vi "报警设置.vi"() -> ()   [LabVIEW 2016, in "环境动力单元.lvlib"]
uses:
  <vilib>/Utility/config.llb/NI_LVConfig.lvlib
panel:
  out "湿度报警解除阈值 %":dbl=90.0
  out "高温报警解除阈值 ℃":dbl=40.0
  out "低压报警解除阈值 V":dbl=13.0
  out "湿度报警阈值 %":dbl=95.0
  out "高温报警阈值 ℃":dbl=50.0
  out "低压报警阈值 V":dbl=11.0
  in  "布尔":bool
  # "参数设置"
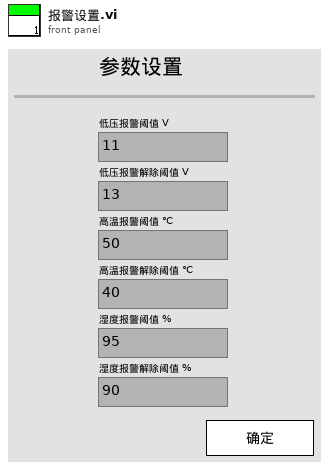
[diagram p1: front panel]
types:
  T1 = cluster{"低压报警阈值 V":dbl, "低压报警解除阈值 V":dbl, "高温报警阈值 ℃":dbl, "高温报警解除阈值 ℃":dbl, "湿度报警阈值 %":dbl, "湿度报警解除阈值 %":dbl}
  T2 = typedef "NI_LVConfig.lvlib/Config Data RefNum.ctl" = refnum<k1>
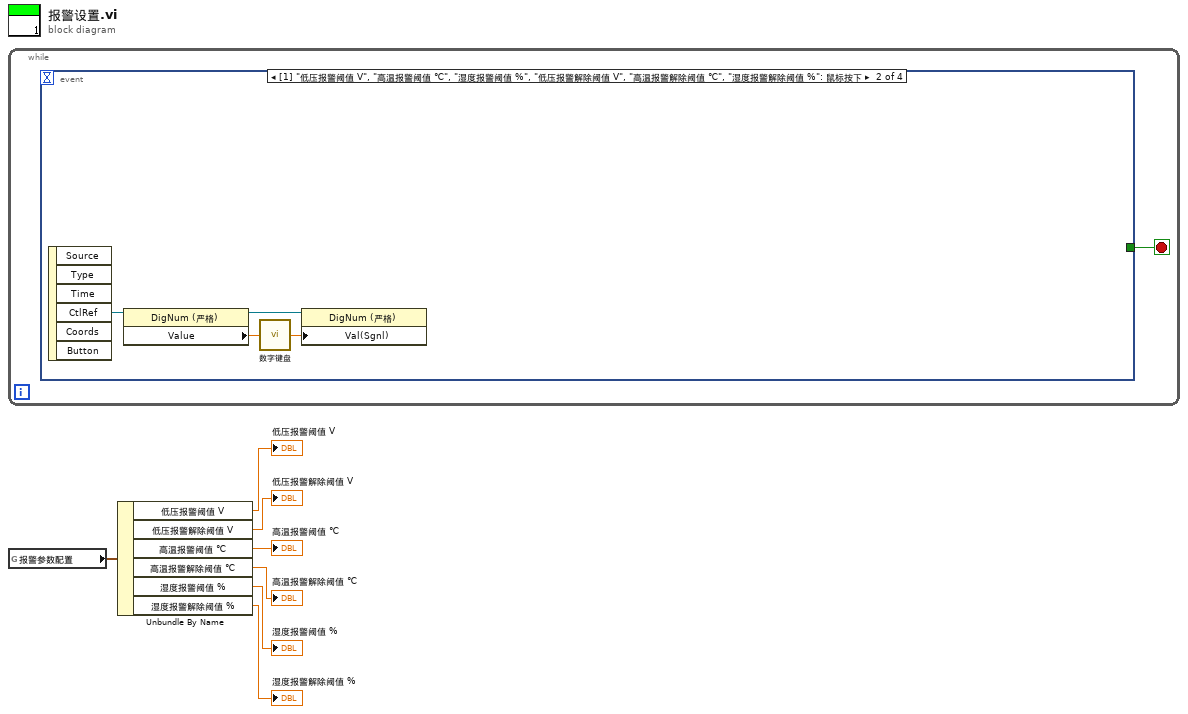
[diagram p0: block diagram]
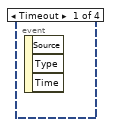
[diagram p2: hidden frame]
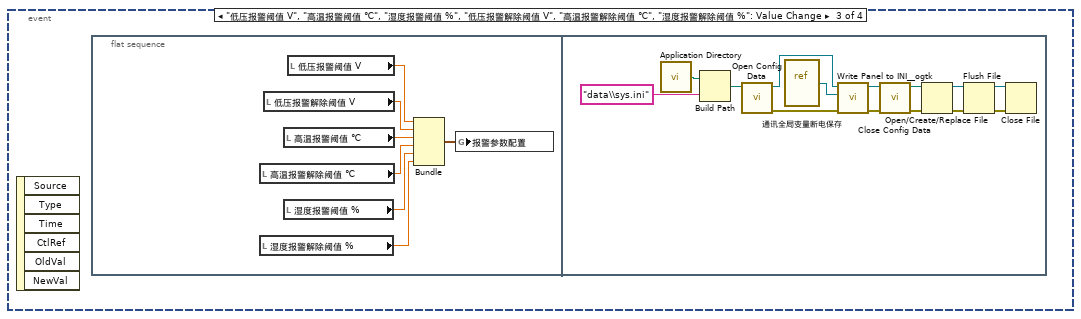
[diagram p3: hidden frame]
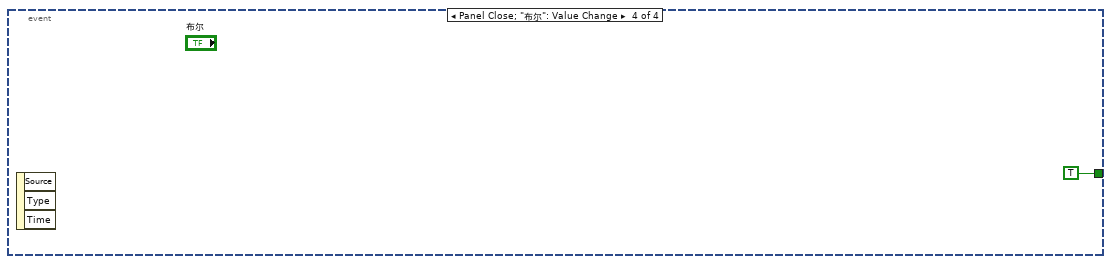
[diagram p4: hidden frame]
diagram:
  n1 = while {
    stop <- w8 stop-if-true
    n2 = event shown="[1] \"低压报警阈值 V\", \"高温报警阈值 ℃\", \"湿度报警阈值 %\", \"低压报警解除阈值 V\", \"高温报警解除阈值 ℃\", \"湿度报警解除阈值 %\": 鼠标按下" {
      selector: _ -> [_ _ _ _]
      dyn-events: _ -> [_ _ _ _]
      timeout: _ -> [_ _ _ _]
      tunnel: [_ _ _ TRUE] -> w8
      event Timeout {
        n3 = event-data() -> ()  [unwired: 1 in, 3 out]
      }
      event "低压报警阈值 V", "高温报警阈值 ℃", "湿度报警阈值 %", "低压报警解除阈值 V", "高温报警解除阈值 ℃", "湿度报警解除阈值 %": Mouse Down {
        n4 = event-data() -> ("CtlRef"=w9:refnum<vi>)  [unwired: 1 in, 5 out]
        n5 = property class="DigNum (严格)"(reference=w9) -> (reference out=w10:refnum<vi>, "Value"=w12:dbl)  [unwired: 1 in, 1 out]
        n6 = call "数字键盘.vi"("OldNumber"=w12) -> ("NewNumber"=w11:dbl)
        n7 = property class="DigNum (严格)"(reference=w10, "Val(Sgnl)"=w11) -> ()  [unwired: 1 in, 2 out]
      }
      event "低压报警阈值 V", "高温报警阈值 ℃", "湿度报警阈值 %", "低压报警解除阈值 V", "高温报警解除阈值 ℃", "湿度报警解除阈值 %": Value Change {
        n8 = event-data() -> ()  [unwired: 1 in, 6 out]
        n9 = flat-sequence {
          frame #0 {
            n10 = local read "高温报警解除阈值 ℃"() -> (w16:dbl)
            n11 = local read "湿度报警解除阈值 %"() -> (w14:dbl)
            n12 = local read "低压报警解除阈值 V"() -> (w18:dbl)
            n13 = local read "高温报警阈值 ℃"() -> (w17:dbl)
            n14 = local read "湿度报警阈值 %"() -> (w15:dbl)
            n15 = local read "低压报警阈值 V"() -> (w19:dbl)
            n16 = Bundle("低压报警阈值 V"=w19, "低压报警解除阈值 V"=w18, "高温报警阈值 ℃"=w17, "高温报警解除阈值 ℃"=w16, "湿度报警阈值 %"=w15, "湿度报警解除阈值 %"=w14) -> (w13:T1)  [unwired: 1 in]
            n17 = global write "通讯全局变量断电保存.vi" "报警参数配置"(w13) -> ()
          }
          frame #1 {
            n18 = call <vilib>:"Application Directory.vi"() -> ("Application Directory"=w33:path)
            n19 = Build Path(base path=w33, name or relative path="data\\sys.ini" ("名称或相对路径")) -> (appended path=w31:path)
            n20 = call <vilib>:"Open Config Data.vi"("configuration file path"=w31) -> ("error out"=w27:errorcluster, "refnum"=w30:T2)  [unwired: 8 in, 1 out]
            n21 = vi-ref "通讯全局变量断电保存.vi"() -> (w29:refnum<vi>)
            n22 = call <userlib>:"Write Panel to INI__ogtk.vi"("error in (no error)"=w27, "VI ref"=w29, "refnum"=w30) -> ("error out"=w26:errorcluster, "refnum out"=w28:T2)  [unwired: 7 in]
            n23 = call <vilib>:"Close Config Data.vi"("error in (no error)"=w26, "refnum"=w28) -> ("error out"=w21:errorcluster, "file path"=w20:path)  [unwired: 8 in]
            n24 = Open/Create/Replace File(file path (use dialog)=w20, error in=w21) -> (refnum out=w24:refnum<file>, error out=w25:errorcluster)  [unwired: 4 in, 1 out]
            n25 = Flush File(refnum=w24, error in=w25) -> (refnum out=w23:refnum<file>, error out=w22:errorcluster)
            n26 = Close File(refnum=w23, error in=w22) -> ()  [unwired: 2 out]
          }
        }
      }
      event Panel Close; "布尔": Value Change {
        n27 = event-data() -> ()  [unwired: 1 in, 3 out]
      }
    }
  }
  n28 = global read "通讯全局变量断电保存.vi" "报警参数配置"() -> (w7:T1)
  n29 = Unbundle By Name(w7) -> ("低压报警阈值 V"=→"低压报警阈值 V":dbl, "低压报警解除阈值 V"=→"低压报警解除阈值 V":dbl, "高温报警阈值 ℃"=→"高温报警阈值 ℃":dbl, "高温报警解除阈值 ℃"=→"高温报警解除阈值 ℃":dbl, "湿度报警阈值 %"=→"湿度报警阈值 %":dbl, "湿度报警解除阈值 %"=→"湿度报警解除阈值 %":dbl)
